vi "begin intake subVI.vi"   [LabVIEW 2017]
uses:
  <vilib>/Rock Robotics/SystemInterfaces/DIO/FPGA_DIOPWMChannel.ctl
  <vilib>/Rock Robotics/WPI/SafetyOutput/WPI_SafetyOutputConfigMenu.ctl
  <vilib>/Rock Robotics/WPI/Solenoid/WPI_SolenoidChannel.ctl
  <vilib>/Rock Robotics/WPI/MotorControl/WPI_MotorControlOpen VictorSP.vi
  <vilib>/Rock Robotics/Network Tables/NT Write Number.vi
  <vilib>/Rock Robotics/WPI/Solenoid/WPI_SolenoidOpenSingle.vi
types:
  T1 = typedef "WPI_SolenoidChannel.ctl" = enum8{"Solenoid 0", "Solenoid 1", "Solenoid 2", "Solenoid 3", "Solenoid 4", "Solenoid 5", "Solenoid 6", "Solenoid 7", "Invalid"}
  T2 = typedef "WPI_SafetyOutputConfigMenu.ctl" = enum16{"Enable", "Disable"}
  T3 = typedef "FPGA_DIOPWMChannel.ctl" = enum8{"PWM 0", "PWM 1", "PWM 2", "PWM 3", "PWM 4", "PWM 5", "PWM 6", "PWM 7", "PWM 8", "PWM 9", "PWM MXP 0", "PWM MXP 1", "PWM MXP 2", "PWM MXP 3", "PWM MXP 4", "PWM MXP 5", "PWM MXP 6", "PWM MXP 7", "PWM MXP 8", "PWM MXP 9", "Invalid"}
  T4 = typedef "WPI_MotorControlDeviceRef.ctl" = cluster{"DeviceStatus":errorcluster, "Type":T5, "PWM":cluster{"PWM Channel":T3, "DeadBand":T6}, "CAN":cluster{"Device Number":u8, "SetOutput VI Ref":variant, "GetOutput VI Ref":variant, "Enable VI Ref":variant, "Disable VI Ref":variant, "Data":variant}, "Invert":bool, "DIO PWM":cluster{"PWM \"Enable\" Channel":T3, "DIOChannel":T7, "PWM Rate":dbl}}
  T5 = typedef "WPI_MotorControlType.ctl" = enum16{"PWM", "CAN", "DIO PWM"}
  T6 = typedef "WPI_PWMDeadband.ctl" = cluster{"Name":string, "maxPositivePwm":i32, "minPositivePwm":i32, "centerPwm":i32, "maxNegativePwm":i32, "minNegativePwm":i32, "angularRange":u16}
  T7 = typedef "FPGA_DIOChannel.ctl" = enum8{"DIO 0", "DIO 1", "DIO 2", "DIO 3", "DIO 4", "DIO 5", "DIO 6", "DIO 7", "DIO 8", "DIO 9", "DIO MXP 0", "DIO MXP 1", "DIO MXP 2", "DIO MXP 3", "DIO MXP 4", "DIO MXP 5", "DIO MXP 6", "DIO MXP 7", "DIO MXP 8", "DIO MXP 9", "DIO MXP 10", "DIO MXP 11", "DIO MXP 12", "DIO MXP 13", "DIO MXP 14", "DIO MXP 15", "SPI Port CS1", "SPI Port CS2", "SPI Port CS3", "SPI Port MISO", "SPI Port MOSI", "Invalid"}
  T8 = typedef "WPI_SolenoidDevRef.ctl" = cluster{"DevStatus":errorcluster, "Pneumatics Control Module":u8, "Forward Solenoid Channel":T1, "Reverse Solenoid Channel":T1}
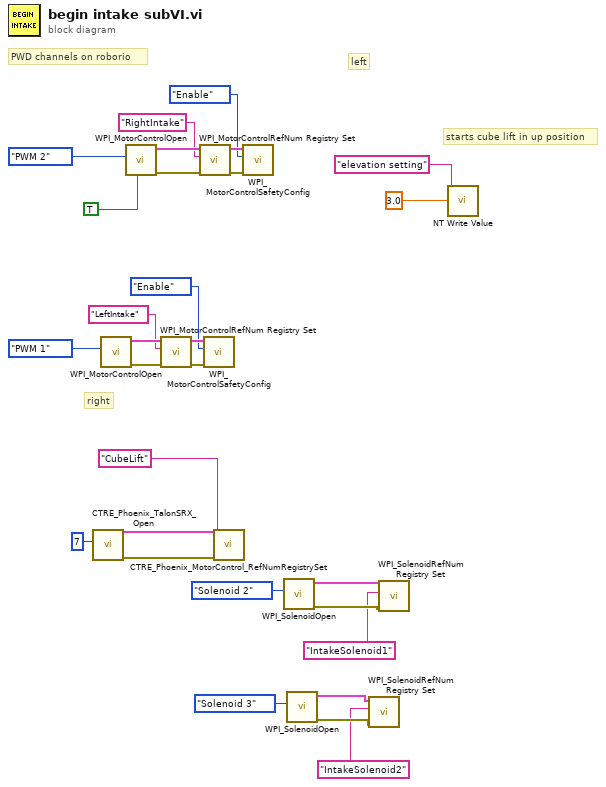
[diagram p0: block diagram]
diagram:
  # "starts cube lift in up position"
  # "right"
  # "left"
  # "PWD channels on roborio"
  n1 = call <vilib>:"CTRE_Phoenix_TalonSRX_Open.vi"("Device Number"=u8 7) -> ("error out"=w10:errorcluster, "CAN Talon SRX Ref"=w11:T4)  [unwired: 9 in]
  n2 = call-poly <vilib>:"WPI_MotorControlOpen.vi"("PWM Channel"=FPGA_DIOPWMChannel."PWM 1") -> ("error out"=w23:errorcluster, "MotorControlDeviceRef"=w25:T4)  [unwired: 9 in]
  n3 = call-poly <vilib>:"WPI_MotorControlOpen.vi"("Invert"=TRUE, "PWM Channel"=FPGA_DIOPWMChannel."PWM 2") -> ("error out"=w24:errorcluster, "MotorControlDeviceRef"=w26:T4)  [unwired: 8 in]
  n4 = call <vilib>:"WPI_MotorControlRefNum Registry Set.vi"("error in (no error)"=w23, "refnum name"="LeftIntake", "MotorControlDevRef"=w25) -> ("error out"=w19:errorcluster, "MotorControlDevRef"=w18:T4)  [unwired: 7 in]
  n5 = call <vilib>:"WPI_MotorControlRefNum Registry Set.vi"("error in (no error)"=w24, "refnum name"="RightIntake", "MotorControlDevRef"=w26) -> ("error out"=w20:errorcluster, "MotorControlDevRef"=w17:T4)  [unwired: 7 in]
  n6 = call <vilib>:"WPI_MotorControlSafetyConfig.vi"("error in (no error)"=w19, "mode"=WPI_SafetyOutputConfigMenu."Enable", "MotorControlDevRef"=w18) -> ()  [unwired: 7 in, 2 out]
  n7 = call <vilib>:"CTRE_Phoenix_MotorControl_RefNumRegistrySet.vi"("error in (no error)"=w10, "refnum name"="CubeLift", "PhoenixMotorControlDevRef"=w11) -> ()  [unwired: 7 in, 2 out]
  n8 = call <vilib>:"WPI_MotorControlSafetyConfig.vi"("error in (no error)"=w20, "mode"=WPI_SafetyOutputConfigMenu."Enable", "MotorControlDevRef"=w17) -> ()  [unwired: 7 in, 2 out]
  n9 = call-poly <vilib>:"WPI_SolenoidOpen.vi"("Solenoid Channel"=WPI_SolenoidChannel."Solenoid 2") -> ("error out"=w7:errorcluster, "SolenoidDevRef"=w8:T8)  [unwired: 9 in]
  n10 = call-poly <vilib>:"WPI_SolenoidOpen.vi"("Solenoid Channel"=WPI_SolenoidChannel."Solenoid 3") -> ("error out"=w5:errorcluster, "SolenoidDevRef"=w6:T8)  [unwired: 9 in]
  n11 = call <vilib>:"WPI_SolenoidRefNum Registry Set.vi"("error in (no error)"=w5, "refnum name"="IntakeSolenoid2", "SolenoidDevRef"=w6) -> ()  [unwired: 7 in, 2 out]
  n12 = call <vilib>:"WPI_SolenoidRefNum Registry Set.vi"("error in (no error)"=w7, "refnum name"="IntakeSolenoid1", "SolenoidDevRef"=w8) -> ()  [unwired: 7 in, 2 out]
  n13 = call-poly <vilib>:"NT Write Value.vi"("Numeric"=3.0, "Name"="elevation setting") -> ()  [unwired: 9 in, 1 out]
